vi "aFGV - Binary File.vi"(6 "State":enum16{"Read", "Write"}(ring)=enum."Write", 8 "Error In":errorcluster, 10 "Path":path, 11 "Data in":variant) -> (0 "Error Out":errorcluster, 3 "Data Out":variant)   [LabVIEW 2020]
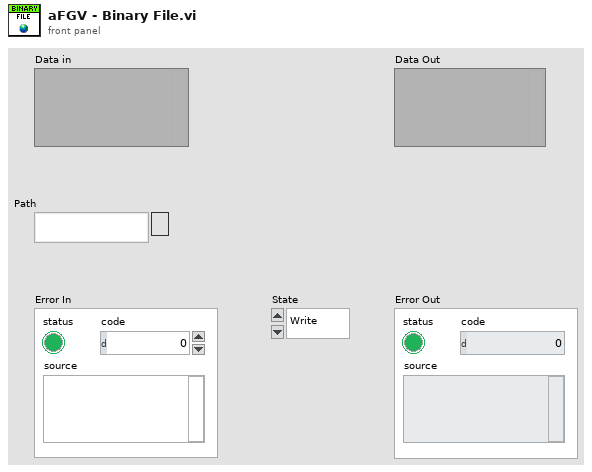
[diagram p1: front panel]
types:
  T1 = enum16{"open", "replace", "create", "open or create", "replace or create", "replace or create with confirmation"}
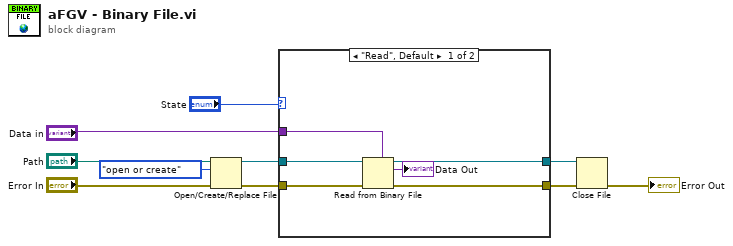
[diagram p0: block diagram]
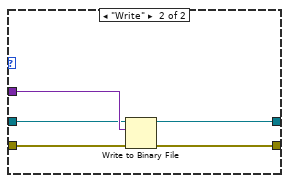
[diagram p2: hidden frame]
diagram:
  n1 = Open/Create/Replace File(file path (use dialog)="Path", error in="Error In", operation (0:open)=T1."open or create") -> (refnum out=w6:refnum<file>, error out=w10:errorcluster)  [unwired: 3 in, 1 out]
  n2 = case shown="\"Read\", Default" "State" {
    tunnel: w10 -> [w16 w21]
    tunnel: [w15 w20] -> w9
    tunnel: w6 -> [w14 w17]
    tunnel: [w13 w19] -> w5
    tunnel: "Data in" -> [w12 w18]
    frame "Read", Default {
      n3 = Read from Binary File(5:w12, 8:w16, 11:w14) -> (0:w15:errorcluster, 2:→"Data Out":variant, 3:w13:refnum<file>)  [unwired: 3 in, 1 out]
    }
    frame "Write" {
      n4 = Write to Binary File(file (use dialog)=w17, data=w18, error in=w21) -> (refnum out=w19:refnum<file>, error out=w20:errorcluster)  [unwired: 3 in, 1 out]
    }
  }
  n5 = Close File(refnum=w5, error in=w9) -> (error out=→"Error Out":errorcluster)  [unwired: 1 out]
